vi "APLUS.vi"(8 "error in (no error)":errorcluster) -> (0 "error out":errorcluster, 2 "Stopped":bool)   [LabVIEW 2019]
uses:
  TypeDef/MB Modbus Command.ctl
  TypeDef/MISURE WT.ctl
  TypeDef/DEVICE NAME.ctl
  <vilib>/Utility/file.llb/Read Delimited Spreadsheet (string).vi
  <vilib>/Modbus/master/Create Master Instance (Serial).vi
  <vilib>/Modbus/master/Modbus Master.lvclass
panel:
  out "# elements in queue":i32
  out "tempo ciclo":u32
  out "element":string
  out "Iteration":i32
  out "STATO":string
  out "MISURE WT":T1
  out "Cluster 2":T2 {"Deviation from average of currents [I1,I2,I3]" format="%.2f"; "Deviation from average of voltages [U1,U2,U3]" format="%.2f"; "Maximum deviation from average of currents" format="%.2f"; "Maximum deviation from average of voltages" format="%.2f"; "Phase angle voltage U3-U1" format="%.2f"; "Phase angle voltage U2-U3" format="%.2f"; "Phase angle voltage U1-U2" format="%.2f"; "Average value of currents (I1+I2+I3)/3" format="%.2f"; "Average value of voltages (U1x+U2x+U3x)/3" format="%.2f"; "Load factor phase 3 (L3 – N)" format="%.2f"; "Load factor phase 2 (L2 – N)" format="%.2f"; "Load factor phase 1 (L1 – N)" format="%.2f"; "sign(Q)·(1 – abs(PF)), Load factor system" format="%.2f"; "Reactive power factor phase 1 (L3 – N)" format="%.2f"; "Reactive power factor phase 1 (L2 – N)" format="%.2f"; "Reactive power factor phase 1 (L1 – N)" format="%.2f"; "QF = Q / S, Reactive power factor system" format="%.2f"; "Power factor phase 3 (L3 – N)" format="%.2f"; "Power factor phase 2 (L2 – N)" format="%.2f"; "Power factor phase 1 (L1 – N)" format="%.2f"; "PF = P / S, Power factor system PF" format="%.2f"; "System frequency" format="%.2f"; "Apparent power phase 3 (L3 – N)" format="%.2f"; "Apparent power phase 2 (L2 – N)" format="%.2f"; "Apparent power phase 1 (L1 – N)" format="%.2f"; "Apparent power system S" format="%.2f"; "Reactive power phase 3 (L3 – N)" format="%.2f"; "Reactive power phase 2 (L2 – N)" format="%.2f"; "Reactive power phase 1 (L1 – N)" format="%.2f"; "Reactive power system (Q = Q1 + Q2 + Q3)" format="%.2f"; "Active power phase 3 (L3 – N)" format="%.2f"; "Active power phase 2 (L2 – N)" format="%.2f"; "Active power phase 1 (L1 – N)" format="%.2f"; "Active power system (P = P1 + P2 + P3)" format="%.2f"; "Bimetal current in phase L3" format="%.2f"; "Bimetal current in phase L2" format="%.2f"; "Bimetal current in phase L 1" format="%.2f"; "Bimet curr in balan load sys" format="%.2f"; "Neutral current" format="%.2f"; "Current in phase L3" format="%.2f"; "Current in phase L2" format="%.2f"; "Current in phase L1" format="%.2f"; "System current" format="%.2f"; "Zero displac volt 4w sys" format="%.2f"; "Voltage phase L3 to L1" format="%.2f"; "Voltage phase L2 to L3" format="%.2f"; "Voltage phase L1 to L2" format="%.2f"; "Voltage phase L3 to N" format="%.2f"; "Voltage phase L2 to N" format="%.2f"; "Voltage phase L1 to N" format="%.2f"; "System voltage" format="%.2f"}
  in  "milliseconds to wait":u32=20
  in  "Tab Control":T3(tab)
  in  "SETUP PORTA SERIALE":T4={"Porta COM"="COM2", "Baud Rate"=19200, "Parity"=0, "Flow Control"=0, "Timeout"=10000, "Mode"=enum."RTU", "Slave Address"=1} {"Flow Control" items=["None", "XON/XOFF", "RTS/CTS", "XON/XOFF & RTS/CTS", "DTR/DSR", "XON/XOFF & DTR/DSR"]; "Parity" items=["None", "Odd", "Even", "Mark", "Space"]}
  out "A primario":dbl format="%.20g"
  out "A secondario":dbl format="%.20g"
  out "Modalità misura":u16
  out "V primario":dbl format="%.20g"
  out "V secondario":dbl format="%.20g"
  out "freq":dbl format="%.20g"
  in  "READ REGISTER":bool
  in  "Modbus Command 2":T5={"Function Code"=3, "Starting Address"=2199, "Quantity"=12, "Data"=[], "Discrete"=[]} {"Function Code" items=["Read Coils"=1, "Read Discrete Inputs"=2, "Read Holding Registers"=3, "Read Input Registers"=4, "Write Single Coil"=5, "Write Single Register"=6, "Read Exception Status"=7, "Write Multiple Coils"=15, "Write Multiple Registers"=16]}
  in  "WRITE MODO MISURA":bool
  in  "Enum":T6(ring)
  in  "PRIM":sgl=20.0 format="%.12f"
  in  "WRITE A PRIM":bool
  in  "SEC":sgl=5.0 format="%.12f"
  in  "WRITE A SEC":bool
  out "Cluster":T7 {"Sys current" format="%.1p"; "Sys voltage" format="%.1p"; "Cosphi" format="%.1p"; "Frequenza" format="%.1p"; "Energia attiva -" format="%.2f"; "Energia attiva +" format="%.2f"; "Tensione FN3" format="%.1p"; "Tensione FN2" format="%.1p"; "Tensione FN1" format="%.1p"; "Papparente" format="%.2f"; "Preattiva" format="%.2f"; "Corrente 3" format="%.3f"; "Corrente 2" format="%.3f"; "TensioneL31" format="%.1p"; "TensioneL23" format="%.1p"; "TensioneL12" format="%.1p"; "Corrente" format="%.3f"; "Pattiva" format="%.2f"}
  out "error in (no error) 2":errorcluster
  # "2199"
  # "12"
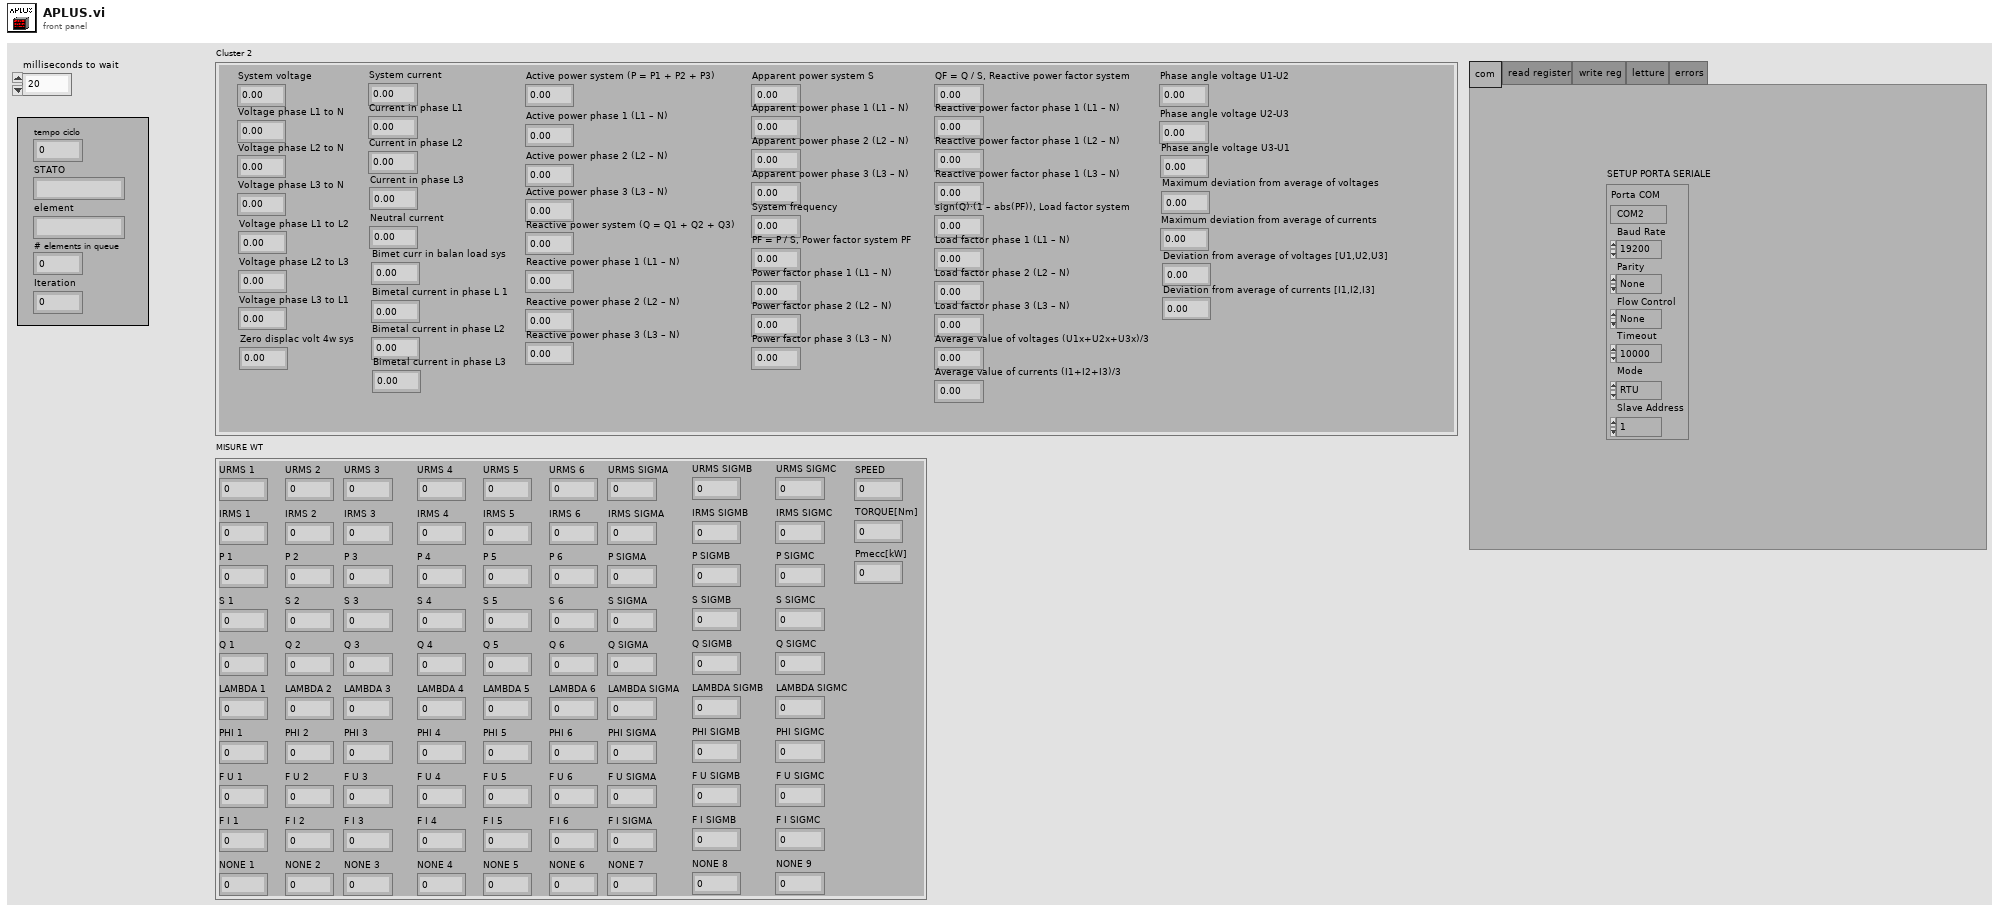
[diagram p1: front panel]
types:
  T1 = typedef "MISURE WT.ctl" = cluster{"URMS 1":dbl, "IRMS 1":dbl, "P 1":dbl, "S 1":dbl, "Q 1":dbl, "LAMBDA 1":dbl, "PHI 1":dbl, "F U 1":dbl, "F I 1":dbl, "NONE 1":dbl, "URMS 2":dbl, "IRMS 2":dbl, "P 2":dbl, "S 2":dbl, "Q 2":dbl, "LAMBDA 2":dbl, "PHI 2":dbl, "F U 2":dbl, "F I 2":dbl, "NONE 2":dbl, "URMS 3":dbl, "IRMS 3":dbl, "P 3":dbl, "S 3":dbl, "Q 3":dbl, "LAMBDA 3":dbl, "PHI 3":dbl, "F U 3":dbl, "F I 3":dbl, "NONE 3":dbl, "URMS 4":dbl, "IRMS 4":dbl, "P 4":dbl, "S 4":dbl, "Q 4":dbl, "LAMBDA 4":dbl, "PHI 4":dbl, "F U 4":dbl, "F I 4":dbl, "NONE 4":dbl, "URMS 5":dbl, "IRMS 5":dbl, "P 5":dbl, "S 5":dbl, "Q 5":dbl, "LAMBDA 5":dbl, "PHI 5":dbl, "F U 5":dbl, "F I 5":dbl, "NONE 5":dbl, "URMS 6":dbl, "IRMS 6":dbl, "P 6":dbl, "S 6":dbl, "Q 6":dbl, "LAMBDA 6":dbl, "PHI 6":dbl, "F U 6":dbl, "F I 6":dbl, "NONE 6":dbl, "URMS SIGMA":dbl, "IRMS SIGMA":dbl, "P SIGMA":dbl, "S SIGMA":dbl, "Q SIGMA":dbl, "LAMBDA SIGMA":dbl, "PHI SIGMA":dbl, "F U SIGMA":dbl, "F I SIGMA":dbl, "NONE 7":dbl, "URMS SIGMB":dbl, "IRMS SIGMB":dbl, "P SIGMB":dbl, "S SIGMB":dbl, "Q SIGMB":dbl, "LAMBDA SIGMB":dbl, "PHI SIGMB":dbl, "F U SIGMB":dbl, "F I SIGMB":dbl, "NONE 8":dbl, "URMS SIGMC":dbl, "IRMS SIGMC":dbl, "P SIGMC":dbl, "S SIGMC":dbl, "Q SIGMC":dbl, "LAMBDA SIGMC":dbl, "PHI SIGMC":dbl, "F U SIGMC":dbl, "F I SIGMC":dbl, "NONE 9":dbl, "SPEED":dbl, "TORQUE[Nm]":dbl, "Pmecc[kW]":dbl}
  T2 = cluster{"System voltage":dbl, "Voltage phase L1 to N":dbl, "Voltage phase L2 to N":dbl, "Voltage phase L3 to N":dbl, "Voltage phase L1 to L2":dbl, "Voltage phase L2 to L3":dbl, "Voltage phase L3 to L1":dbl, "Zero displac volt 4w sys":dbl, "System current":dbl, "Current in phase L1":dbl, "Current in phase L2":dbl, "Current in phase L3":dbl, "Neutral current":dbl, "Bimet curr in balan load sys":dbl, "Bimetal current in phase L 1":dbl, "Bimetal current in phase L2":dbl, "Bimetal current in phase L3":dbl, "Active power system (P = P1 + P2 + P3)":dbl, "Active power phase 1 (L1 – N)":dbl, "Active power phase 2 (L2 – N)":dbl, "Active power phase 3 (L3 – N)":dbl, "Reactive power system (Q = Q1 + Q2 + Q3)":dbl, "Reactive power phase 1 (L1 – N)":dbl, "Reactive power phase 2 (L2 – N)":dbl, "Reactive power phase 3 (L3 – N)":dbl, "Apparent power system S":dbl, "Apparent power phase 1 (L1 – N)":dbl, "Apparent power phase 2 (L2 – N)":dbl, "Apparent power phase 3 (L3 – N)":dbl, "System frequency":dbl, "PF = P / S, Power factor system PF":dbl, "Power factor phase 1 (L1 – N)":dbl, "Power factor phase 2 (L2 – N)":dbl, "Power factor phase 3 (L3 – N)":dbl, "QF = Q / S, Reactive power factor system":dbl, "Reactive power factor phase 1 (L1 – N)":dbl, "Reactive power factor phase 1 (L2 – N)":dbl, "Reactive power factor phase 1 (L3 – N)":dbl, "sign(Q)·(1 – abs(PF)), Load factor system":dbl, "Load factor phase 1 (L1 – N)":dbl, "Load factor phase 2 (L2 – N)":dbl, "Load factor phase 3 (L3 – N)":dbl, "Average value of voltages (U1x+U2x+U3x)/3":dbl, "Average value of currents (I1+I2+I3)/3":dbl, "Phase angle voltage U1-U2":dbl, "Phase angle voltage U2-U3":dbl, "Phase angle voltage U3-U1":dbl, "Maximum deviation from average of voltages":dbl, "Maximum deviation from average of currents":dbl, "Deviation from average of voltages [U1,U2,U3]":dbl, "Deviation from average of currents [I1,I2,I3]":dbl}
  T3 = enum32{"com", "read register", "write reg", "letture", "errors"}
  T4 = cluster{"Porta COM":string, "Baud Rate":u32, "Parity":u16, "Flow Control":u16, "Timeout":u32, "Mode":enum16{"RTU", "ASCII"}, "Slave Address":u8}
  T5 = typedef "MB Modbus Command.ctl" = cluster{"Function Code":u8, "Starting Address":u16, "Quantity":u16, "Data":u16[], "Discrete":bool[]}
  T6 = enum16{"SINGLE PH", "SPLIT PHASE", "3W,B", "3W,B,U12", "3W,B,U23", "3W,B,U31", "3W,U", "3W,U,ARON", "4W,B", "4W,U", "4W,U,OPEN_Y"}
  T7 = cluster{"Pattiva":dbl, "Corrente":dbl, "TensioneL12":dbl, "TensioneL23":dbl, "TensioneL31":dbl, "Corrente 2":dbl, "Corrente 3":dbl, "Preattiva":dbl, "Papparente":dbl, "Tensione FN1":dbl, "Tensione FN2":dbl, "Tensione FN3":dbl, "Energia attiva +":dbl, "Energia attiva -":dbl, "Frequenza":dbl, "Cosphi":dbl, "Sys voltage":dbl, "Sys current":dbl}
  T8 = typedef "DEVICE NAME.ctl" = enum16{"WATTMETRO", "APLUS", "PLC BANCO 1", "PLC RACK", "PLC BANCO 2", "PS", "NI cDAQ", "RESISTOMAT"}
  T9 = cluster{"Array of elements":cluster{"String":string, "variant":variant}[], "Single element":cluster{"String":string, "variant":variant}, "enque at\nopposite end (F)":bool, "no replications (F)":bool}
  T10 = enum16{"ALIGN -CENTER", "ALIGN -TOP LEFT", "ALIGN -AS IS", "ALIGN -CUSTOM"}
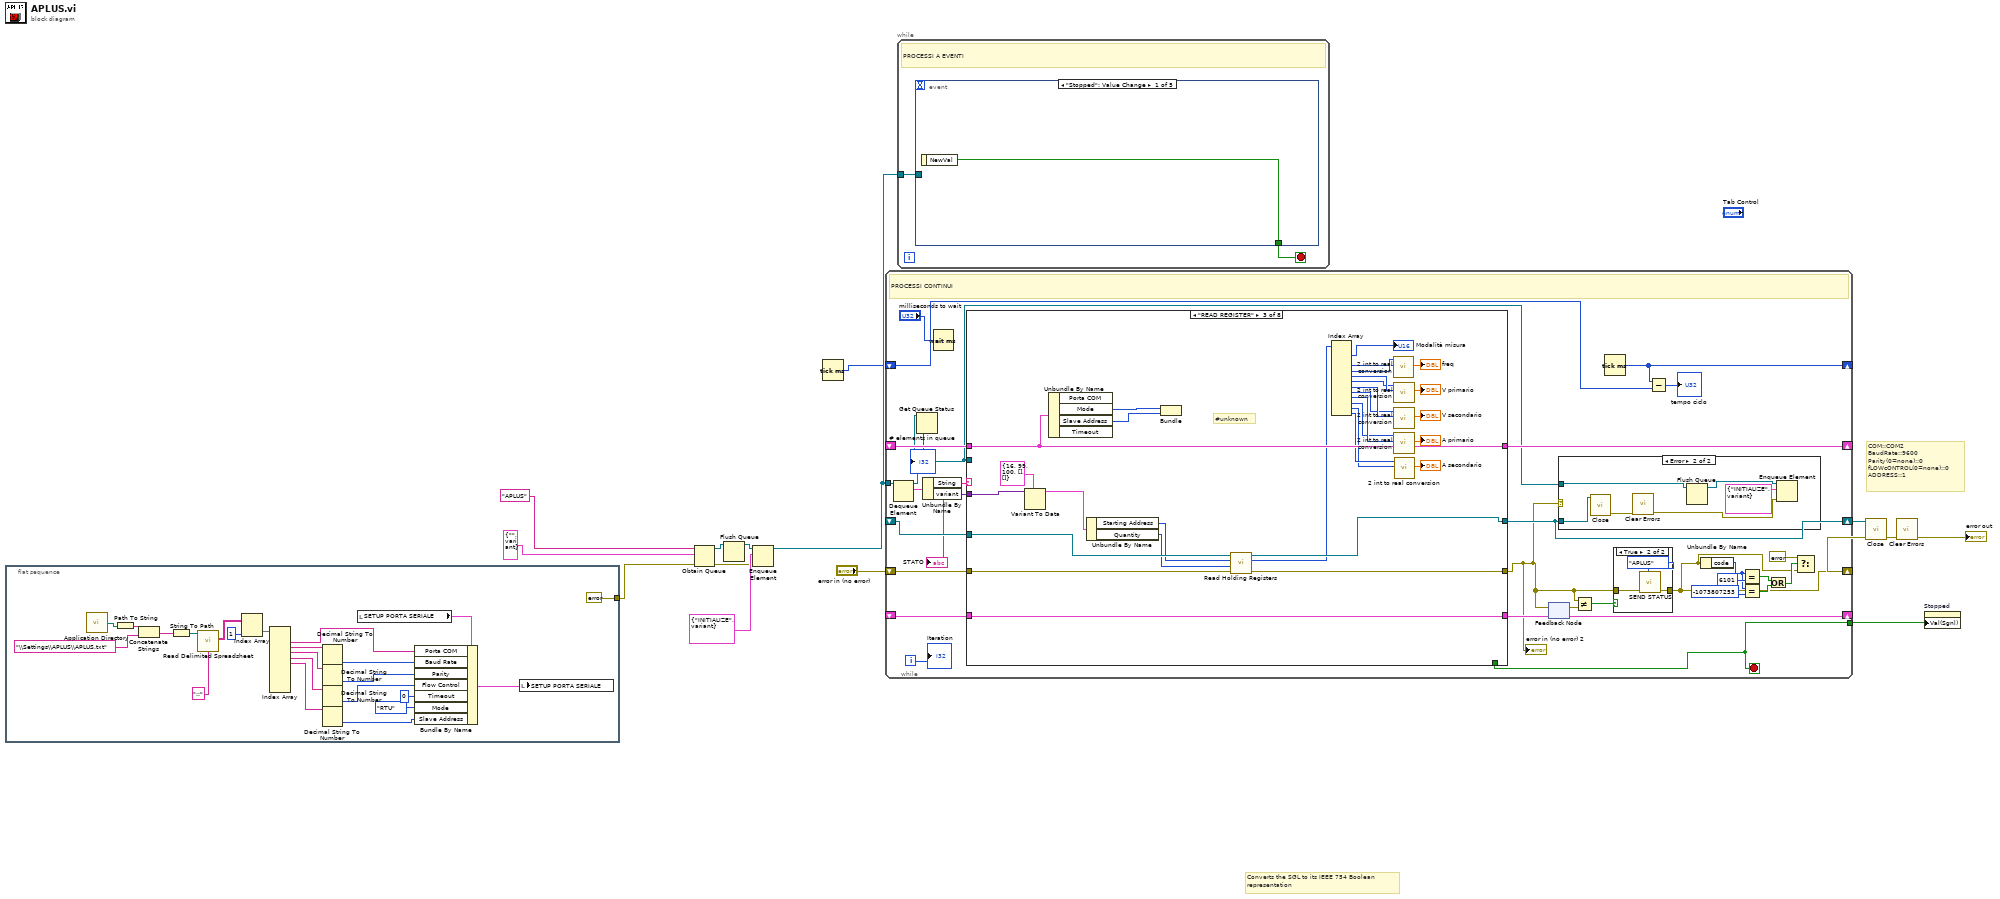
[diagram p0: block diagram]
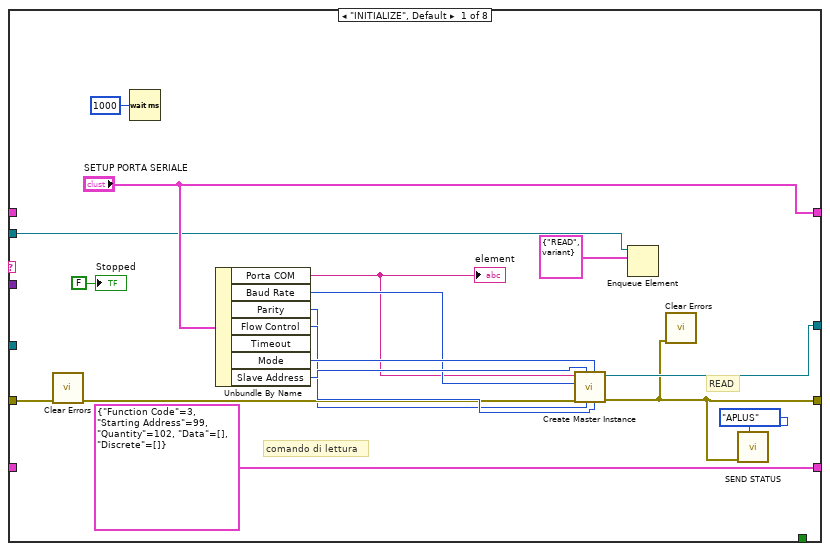
[diagram p4: hidden frame]
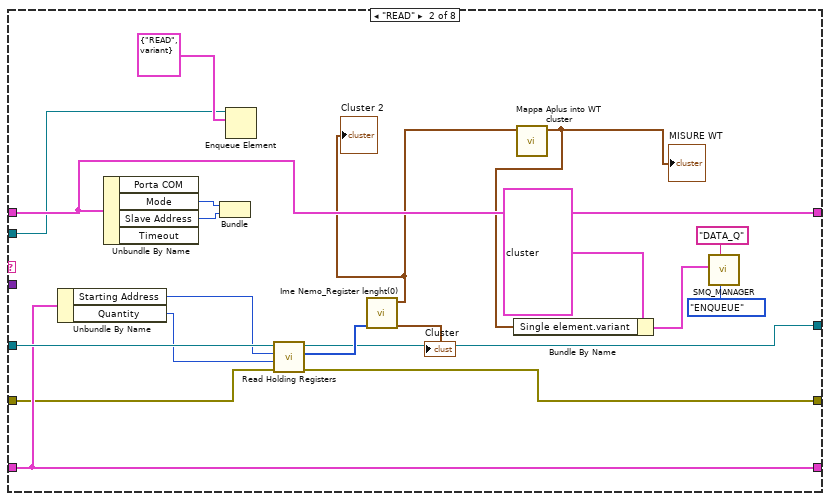
[diagram p5: hidden frame]
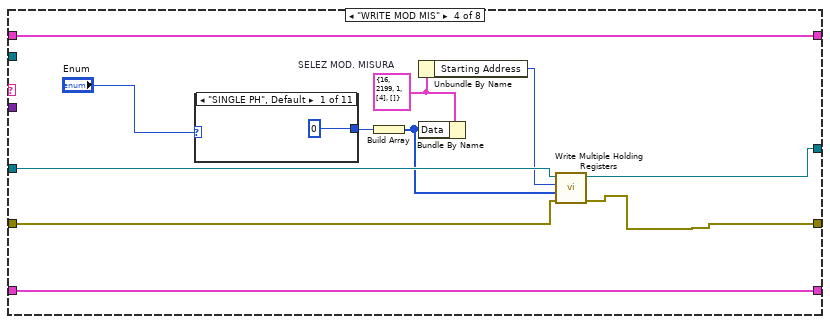
[diagram p6: hidden frame]
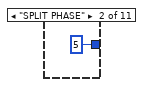
[diagram p7: hidden frame]
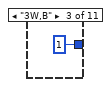
[diagram p8: hidden frame]
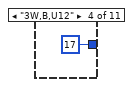
[diagram p9: hidden frame]
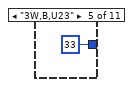
[diagram p10: hidden frame]
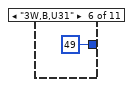
[diagram p11: hidden frame]
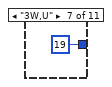
[diagram p12: hidden frame]
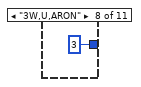
[diagram p13: hidden frame]
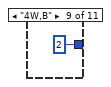
[diagram p14: hidden frame]
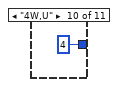
[diagram p15: hidden frame]
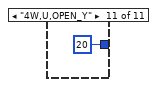
[diagram p16: hidden frame]
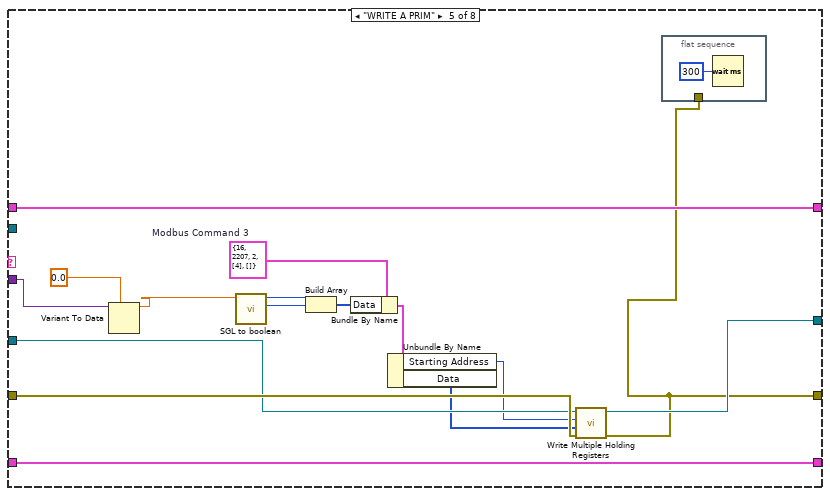
[diagram p17: hidden frame]
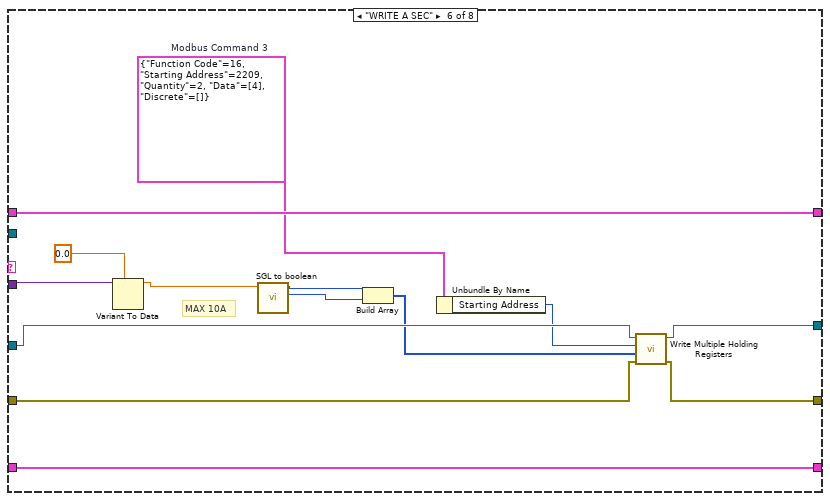
[diagram p18: hidden frame]
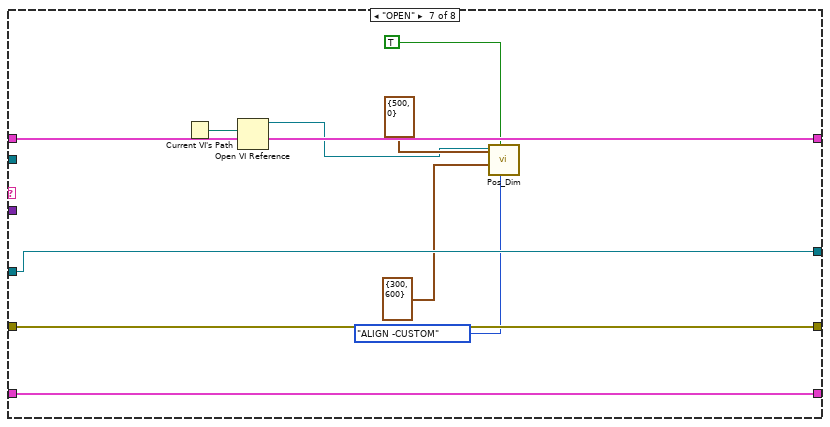
[diagram p19: hidden frame]
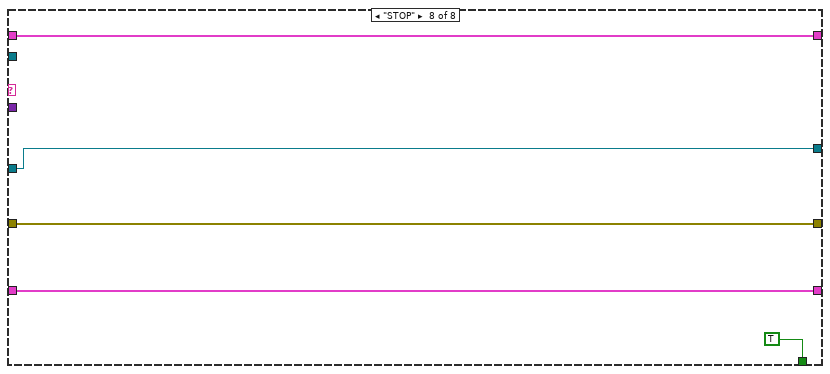
[diagram p20: hidden frame]
diagram:
  # "COM::COM2\nBaudRate::9600\nParity(0=none)::0\nfLOWcONTROL(0=none)::0\nADDRESS::1"
  # "Converts the SGL to its IEEE 754 Boolean \nrepresentation"
  n1 = flat-sequence {
    tunnel: [errorcluster {"status"=FALSE, "code"=0, "source"=""} ("error out")] -> w2
    frame #0 {
      n2 = call <vilib>:"Application Directory.vi"() -> ("Application Directory"=w26:path)
      n3 = Path To String(path=w26) -> (string=w27:string)
      n4 = Concatenate Strings(w27, "\\Settings\\APLUS\\APLUS.txt" ("string")) -> (w29:string)
      n5 = String To Path(string=w29) -> (path=w30:path)
      n6 = call-poly <vilib>:"Read Delimited Spreadsheet.vi"("file path (dialog if empty)"=w30, "delimiter (\\t)"="::" ("delimiter (\\t)")) -> ("all rows"=w31:string[][])  [unwired: 8 in, 5 out]
      n7 = Index Array(array=w31, index (col)=1 ("disabled index (col)")) -> (element=w33:string[])  [unwired: 1 in]
      n8 = Index Array(array=w33) -> (element #1=w22:string, element #2=w34:string, element #3=w35:string, element #4=w36:string, element #5=w37:string)  [unwired: 10 in, 5 out]
      n9 = Decimal String To Number(string=w34) -> (number=w21:i32)  [unwired: 2 in, 1 out]
      n10 = Decimal String To Number(string=w35) -> (number=w20:i32)  [unwired: 2 in, 1 out]
      n11 = Decimal String To Number(string=w36) -> (number=w19:i32)  [unwired: 2 in, 1 out]
      n12 = Decimal String To Number(string=w37) -> (number=w17:i32)  [unwired: 2 in, 1 out]
      n13 = local read "SETUP PORTA SERIALE"() -> (w24:T4)
      n14 = Bundle By Name(cluster=w24, "Porta COM"=w22, "Baud Rate"=w21, "Parity"=w20, "Flow Control"=w19, "Timeout"=u32 0, "Mode"=enum16{"RTU", "ASCII"}."RTU", "Slave Address"=w17) -> (w23:T4)
      n15 = local write "SETUP PORTA SERIALE"(w23) -> ()
    }
  }
  n16 = Obtain Queue(name (unnamed)="APLUS", element data type=cluster{"String":string, "variant":variant} {"String"="", "variant"=variant} ("element"), error in (no error)=w2) -> (queue out=w4:refnum<queue>, error out=w6:errorcluster)  [unwired: 2 in, 1 out]
  n17 = Flush Queue(queue=w4) -> (queue out=w3:refnum<queue>)  [unwired: 1 in, 2 out]
  n18 = Enqueue Element(queue=w3, element=cluster{"String":string, "variant":variant} {"String"="INITIALIZE", "variant"=variant}, error in (no error)=w6) -> (queue out=w13:refnum<queue>)  [unwired: 1 in, 2 out]
  n19 = Tick Count (ms)() -> (millisecond timer value=w1:u32)
  n20 = while {
    shift-right: [w47] -> w11
    shift-left: "error in (no error)" -> [w68]
    tunnel: w13 -> [w52]
    tunnel: [w48] -> w14
    shift-right: [w54] -> _
    shift-left: _ -> [w66]
    shift-right: [w65] -> _
    shift-left: _ -> [w64]
    shift-right: [w53] -> w12
    shift-left: _ -> [w55]
    shift-right: [w46] -> _
    shift-left: w1 -> [w45]
    i -> [w63]
    stop <- w48 stop-if-true
    # "PROCESSI CONTINUI"
    n21 = Dequeue Element(queue=w52) -> (queue out=w43:refnum<queue>, element=w51:cluster{"String":string, "variant":variant})  [unwired: 2 in, 2 out]
    n22 = Get Queue Status(queue=w43) -> (# elements in queue=→"# elements in queue":i32)  [unwired: 2 in, 7 out]
    n23 = Unbundle By Name(w51) -> ("String"=w49:string, "variant"=w50:variant)
    "STATO" <- w49
    n24 = Wait (ms)(milliseconds to wait="milliseconds to wait") -> ()  [unwired: 1 out]
    n25 = case shown="\"READ REGISTER\"" w49 {
      tunnel: [_ _ _ _ _ _ _ TRUE] -> w48
      tunnel: w68 -> [w84 w105 w123 w153 w177 w194 w208 w212]
      tunnel: [w79 w104 w122 w147 w171 w193 w208 w212] -> w40
      tunnel: w50 -> [_ _ w144 _ w170 w186 _ _]
      tunnel: w64 -> [_ w108 w145 w156 w183 w198 w206 w210]
      tunnel: ["SETUP PORTA SERIALE" w115 w140 w155 w181 w197 w207 w211] -> w54
      tunnel: w66 -> [_ w115 w140 w155 w181 w197 w207 w211]
      tunnel: [T5 {"Function Code"=3, "Starting Address"=99, "Quantity"=102, "Data"=[], "Discrete"=[]} ("Modbus Command") w108 w145 w156 w183 w198 w206 w210] -> w65
      tunnel: w43 -> [w91 w111 _ _ _ _ _ _]
      tunnel: [w85 w106 w120 w151 w175 w191 w205 w209] -> w53
      tunnel: w55 -> [_ w109 w121 w152 w176 w192 w205 w209]
      frame "INITIALIZE", Default {
        # "comando di lettura"
        # "READ"
        n26 = call <vilib>:"Clear Errors.vi"("error in (no error)"=w84) -> ("error out"=w83:errorcluster)  [unwired: 5 in, 1 out]
        n27 = Wait (ms)(milliseconds to wait=u32 1000) -> ()  [unwired: 1 out]
        n28 = Unbundle By Name("SETUP PORTA SERIALE") -> ("Porta COM"=w82:string, "Baud Rate"=w87:u32, "Parity"=w81:u16, "Flow Control"=w86:u16, "Mode"=w88:enum16{"RTU", "ASCII"}, "Slave Address"=w89:u8)  [unwired: 1 out]
        "element" <- w82
        n29 = call-poly <vilib>:"Create Master Instance.vi"("flow control (None)"=w86, "serial type"=w88, "parity (Even)"=w81, "unit ID"=w89, "error in (no error)"=w83, "baud rate (9600)"=w87, "VISA resource name"=w82) -> ("error out"=w79:errorcluster, "serial master instance"=w85:refnum<class "Modbus Master.lvclass">)  [unwired: 3 in]
        n30 = Enqueue Element(queue=w91, element=cluster{"String":string, "variant":variant} {"String"="READ", "variant"=variant}) -> ()  [unwired: 2 in, 3 out]
        n31 = call <vilib>:"Clear Errors.vi"("error in (no error)"=w79) -> ()  [unwired: 5 in, 2 out]
        n32 = call "SEND STATUS.vi"("ELEMENT"=DEVICE_NAME."APLUS", "error in (no error)"=w79) -> ()  [unwired: 9 in, 1 out]
        "Stopped" <- FALSE ("Stop")
      }
      frame "READ" {
        n33 = Unbundle By Name(w108) -> ("Starting Address"=w103:u16, "Quantity"=w102:u16)
        n34 = Unbundle By Name(w115) -> ("Mode"=w114:enum16{"RTU", "ASCII"}, "Slave Address"=w113:u8)  [unwired: 2 out]
        n35 = Bundle("Mode"=w114, "Slave Address"=w113) -> ()  [unwired: 1 in, 1 out]
        n36 = Enqueue Element(queue=w111, element=cluster{"String":string, "variant":variant} {"String"="READ", "variant"=variant}) -> ()  [unwired: 2 in, 3 out]
        n37 = call-dynamic "Read Holding Registers.vi"("error in (no error)"=w105, "number of holding registers"=w102, "starting address"=w103, "Modbus master in"=w109) -> ("error out"=w104:errorcluster, "register values"=w107:u16[], "Modbus master out"=w106:refnum<class "Modbus Master.lvclass">)  [unwired: 5 in]
        n38 = call "Ime Nemo_Register lenght(0).vi"("Array U16"=w107) -> ("Cluster"=→"Cluster":T7, "Cluster 2"=w101:T2)  [unwired: 9 in]
        "Cluster 2" <- w101
        n39 = call "Mappa Aplus into WT cluster.vi"("Cluster in"=w101) -> ("MISURE WT"=w96:T1)  [unwired: 10 in]
        "MISURE WT" <- w96
        n40 = Bundle By Name(cluster=T9 {"Array of elements"=[], "Single element"={"String"="READ WT", "variant"=variant}, "enque at\nopposite end (F)"=FALSE, "no replications (F)"=FALSE} ("Enqueue cluster"), "Single element.variant"=w96) -> (w97:T9)
        n41 = call <userlib>:"SMQ_MANAGER.vi"("Function"=enum16{"INITIALIZE", "ENQUEUE", "STOP ALL"}."ENQUEUE", "Queue name"="DATA_Q", "Enqueue cluster"=w97) -> ()  [unwired: 8 in, 1 out]
      }
      frame "READ REGISTER" {
        # "#unknown"
        n42 = Variant To Data(type=T5 {"Function Code"=16, "Starting Address"=99, "Quantity"=100, "Data"=[], "Discrete"=[]} ("Modbus Command"), Variant=w144) -> (data=w119:T5)  [unwired: 1 in, 1 out]
        n43 = Unbundle By Name(w140) -> ("Mode"=w142:enum16{"RTU", "ASCII"}, "Slave Address"=w141:u8)  [unwired: 2 out]
        n44 = Unbundle By Name(w119) -> ("Starting Address"=w118:u16, "Quantity"=w117:u16)
        n45 = Bundle("Mode"=w142, "Slave Address"=w141) -> ()  [unwired: 1 in, 1 out]
        n46 = call-dynamic "Read Holding Registers.vi"("error in (no error)"=w123, "number of holding registers"=w117, "starting address"=w118, "Modbus master in"=w121) -> ("error out"=w122:errorcluster, "register values"=w116:u16[], "Modbus master out"=w120:refnum<class "Modbus Master.lvclass">)  [unwired: 5 in]
        n47 = Index Array(array=w116) -> (element #1=→"Modalità misura":u16, element #3=w124:u16, element #4=w125:u16, element #5=w129:u16, element #6=w128:u16, element #7=w136:u16, element #8=w135:u16, element #9=w133:u16, element #10=w132:u16, element #11=w130:u16, element #12=w131:u16)  [unwired: 12 in, 1 out]
        n48 = call "2 int to real conversion.vi"("MW 15 0 in"=w124, "MW 31 16 in"=w125) -> ("reale out"=→"freq":dbl)  [unwired: 7 in, 2 out]
        n49 = call "2 int to real conversion.vi"("MW 15 0 in"=w129, "MW 31 16 in"=w128) -> ("reale out"=→"V primario":dbl)  [unwired: 7 in, 2 out]
        n50 = call "2 int to real conversion.vi"("MW 15 0 in"=w136, "MW 31 16 in"=w135) -> ("reale out"=→"V secondario":dbl)  [unwired: 7 in, 2 out]
        n51 = call "2 int to real conversion.vi"("MW 15 0 in"=w133, "MW 31 16 in"=w132) -> ("reale out"=→"A primario":dbl)  [unwired: 7 in, 2 out]
        n52 = call "2 int to real conversion.vi"("MW 15 0 in"=w130, "MW 31 16 in"=w131) -> ("reale out"=→"A secondario":dbl)  [unwired: 7 in, 2 out]
      }
      frame "WRITE MOD MIS" {
        w149 = T5 {"Function Code"=16, "Starting Address"=2199, "Quantity"=1, "Data"=[4], "Discrete"=[]}  # SELEZ MOD. MISURA
        n53 = case shown="\"SINGLE PH\", Default" "Enum" {
          tunnel: [i8 0 ("Numeric 2") i8 5 ("Numeric 2") i8 1 ("Numeric 2") i8 17 ("Numeric 2") i8 33 ("Numeric 2") i8 49 ("Numeric 2") i8 19 ("Numeric 2") i8 3 ("Numeric 2") i8 2 ("Numeric 2") i8 4 ("Numeric 2") i8 20 ("Numeric 2")] -> w154
          frame "SINGLE PH", Default {
          }
          frame "SPLIT PHASE" {
          }
          frame "3W,B" {
          }
          frame "3W,B,U12" {
          }
          frame "3W,B,U23" {
          }
          frame "3W,B,U31" {
          }
          frame "3W,U" {
          }
          frame "3W,U,ARON" {
          }
          frame "4W,B" {
          }
          frame "4W,U" {
          }
          frame "4W,U,OPEN_Y" {
          }
        }
        n54 = Build Array(w154) -> (w150:i8[])
        n55 = Unbundle By Name(w149) -> ("Starting Address"=w148:u16)
        n56 = Bundle By Name(cluster=w149, "Data"=w150) -> ()  [unwired: 1 out]
        n57 = call-dynamic "Write Multiple Holding Registers.vi"("error in (no error)"=w153, "holding register values"=w150, "starting address"=w148, "Modbus master in"=w152) -> ("error out"=w147:errorcluster, "Modbus master out"=w151:refnum<class "Modbus Master.lvclass">)  [unwired: 6 in]
      }
      frame "WRITE A PRIM" {
        w178 = T5 {"Function Code"=16, "Starting Address"=2207, "Quantity"=2, "Data"=[4], "Discrete"=[]}  # Modbus Command 3
        n58 = Variant To Data(type=0.0, Variant=w170) -> (data=w169:dbl)  [unwired: 1 in, 1 out]
        n59 = call "SGL to boolean.vi"("Number"=w169) -> ("Numeric 2"=w179:u32, "Numeric"=w180:u32)  [unwired: 9 in]
        n60 = Build Array(w180, w179) -> (w182:u32[])
        n61 = Bundle By Name(cluster=w178, "Data"=w182) -> (w174:T5)
        n62 = Unbundle By Name(w174) -> ("Starting Address"=w173:u16, "Data"=w172:u16[])
        n63 = call-dynamic "Write Multiple Holding Registers.vi"("error in (no error)"=w177, "holding register values"=w172, "starting address"=w173, "Modbus master in"=w176) -> ("error out"=w171:errorcluster, "Modbus master out"=w175:refnum<class "Modbus Master.lvclass">)  [unwired: 6 in]
        n64 = flat-sequence {
          tunnel: w171 -> [_]
          frame #0 {
            n65 = Wait (ms)(milliseconds to wait=u32 300) -> ()  [unwired: 1 out]
          }
        }
      }
      frame "WRITE A SEC" {
        w189 = T5 {"Function Code"=16, "Starting Address"=2209, "Quantity"=2, "Data"=[4], "Discrete"=[]}  # Modbus Command 3
        # "MAX 10A"
        n66 = Variant To Data(type=0.0, Variant=w186) -> (data=w185:dbl)  [unwired: 1 in, 1 out]
        n67 = call "SGL to boolean.vi"("Number"=w185) -> ("Numeric 2"=w195:u32, "Numeric"=w196:u32)  [unwired: 9 in]
        n68 = Build Array(w196, w195) -> (w190:u32[])
        n69 = Unbundle By Name(w189) -> ("Starting Address"=w188:u16)
        n70 = call-dynamic "Write Multiple Holding Registers.vi"("error in (no error)"=w194, "holding register values"=w190, "starting address"=w188, "Modbus master in"=w192) -> ("error out"=w193:errorcluster, "Modbus master out"=w191:refnum<class "Modbus Master.lvclass">)  [unwired: 6 in]
      }
      frame "OPEN" {
        n71 = Current VI's Path() -> (path=w200:path)
        n72 = Open VI Reference(vi path=w200) -> (vi reference=w199:refnum<vi>)  [unwired: 1 in, 5 out]
        n73 = call "Pos_Dim.vi"("Mode"=T10."ALIGN -CUSTOM", "Open FP"=TRUE, "Size"=cluster{"right":i16, "bottom":i16} {"right"=300, "bottom"=600}, "Poistion"=cluster{"left":i16, "top":i16} {"left"=500, "top"=0}, "VIRefNum  IN"=w199) -> ()  [unwired: 2 in, 5 out]
      }
      frame "STOP" {
      }
    }
    "error in (no error) 2" <- w40
    n74 = feedback-in #1(w40) -> ()
    n75 = feedback #1() -> (w41:errorcluster)  [unwired: 1 in]
    n76 = case shown="Error" w40 {
      tunnel: w43 -> [_ w74]
      tunnel: w53 -> [_ w78]
      frame No Error {
      }
      frame Error {
        n77 = call-dynamic "Close.vi"("Modbus master in"=w78) -> ("error out"=w76:errorcluster)  [unwired: 10 in]
        n78 = call <vilib>:"Clear Errors.vi"("error in (no error)"=w76) -> ("error out"=w75:errorcluster)  [unwired: 5 in, 1 out]
        n79 = Flush Queue(queue=w74) -> (queue out=w73:refnum<queue>)  [unwired: 1 in, 2 out]
        n80 = Enqueue Element(queue=w73, element=cluster{"String":string, "variant":variant} {"String"="INITIALIZE", "variant"=variant}, error in (no error)=w75) -> ()  [unwired: 1 in, 3 out]
      }
    }
    n81 = Not Equal?(x=w40, y=w41) -> (x != y?=w39:bool)
    n82 = Tick Count (ms)() -> (millisecond timer value=w46:u32)
    n83 = case shown="True" w39 {
      tunnel: [w69 w71] -> w47
      tunnel: w40 -> [w69 w70]
      frame False {
      }
      frame True {
        n84 = call "SEND STATUS.vi"("ELEMENT"=DEVICE_NAME."APLUS", "error in (no error)"=w70) -> ("error out"=w71:errorcluster)  [unwired: 9 in]
      }
    }
    n85 = Subtract(x=w46, y=w45) -> (x-y=→"tempo ciclo":u32)
    n86 = Unbundle By Name(w47) -> ("code"=w59:i32)
    n87 = Equal?(x=w59, y=6101) -> (x = y?=w60:bool)
    n88 = Equal?(x=w59, y=-1073807253) -> (x = y?=w57:bool)
    n89 = Or(x=w60, y=w57) -> (x .or. y?=w56:bool)
    n90 = Select(t=errorcluster {"status"=FALSE, "code"=0, "source"=""}, s=w56, f=w47) -> ()  [unwired: 1 out]
    "Iteration" <- w63
  }
  n91 = while {
    tunnel: w13 -> [w214]
    stop <- w215 stop-if-true
    # "PROCESSI A EVENTI"
    n92 = event shown="[0] \"Stopped\": Value Change" {
      selector: _ -> [_ _ _ _ _]
      dyn-events: _ -> [_ _ _ _ _]
      timeout: _ -> [_ _ _ _ _]
      tunnel: [w216 _ _ _ _] -> w215
      tunnel: w214 -> [_ w217 w224 w228 w235]
      event "Stopped": Value Change {
        n93 = event-data() -> ("NewVal"=w216:bool)  [unwired: 1 in]
      }
      event "READ REGISTER": Value Change {
        n94 = event-data() -> ("NewVal"=w218:bool)  [unwired: 1 in]
        n95 = case shown="True" w218 {
          tunnel: w217 -> [_ w223]
          frame False {
          }
          frame True {
            n96 = To Variant(anything="Modbus Command 2") -> (Variant=w220:variant)
            n97 = Bundle By Name(cluster=cluster{"String":string, "variant":variant} {"String"="READ REGISTER", "variant"=variant} ("element"), "variant"=w220) -> (w219:cluster{"String":string, "variant":variant})
            n98 = Enqueue Element(queue=w223, element=w219) -> ()  [unwired: 2 in, 3 out]
          }
        }
      }
      event "WRITE MODO MISURA": Value Change {
        n99 = event-data() -> ("NewVal"=w225:bool)  [unwired: 1 in, 1 out]
        n100 = case shown="True" w225 {
          tunnel: w224 -> [_ w227]
          frame False {
          }
          frame True {
            n101 = Enqueue Element(queue=w227, element=cluster{"String":string, "variant":variant} {"String"="WRITE MOD MIS", "variant"=variant}) -> ()  [unwired: 2 in, 3 out]
          }
        }
      }
      event "WRITE A PRIM": Value Change {
        n102 = event-data() -> ("NewVal"=w229:bool)  [unwired: 1 in, 1 out]
        n103 = case shown="True" w229 {
          tunnel: w228 -> [_ w233]
          frame False {
          }
          frame True {
            n104 = Bundle By Name(cluster=cluster{"String":string, "variant":variant} {"String"="WRITE A PRIM", "variant"=variant} ("element"), "variant"="PRIM") -> (w231:cluster{"String":string, "variant":variant})
            n105 = Enqueue Element(queue=w233, element=w231) -> ()  [unwired: 2 in, 3 out]
          }
        }
      }
      event "WRITE A SEC": Value Change {
        n106 = event-data() -> ("NewVal"=w234:bool)  [unwired: 1 in, 1 out]
        n107 = case shown="True" w234 {
          tunnel: w235 -> [_ w239]
          frame False {
          }
          frame True {
            n108 = Bundle By Name(cluster=cluster{"String":string, "variant":variant} {"String"="WRITE A SEC", "variant"=variant} ("element"), "variant"="SEC") -> (w237:cluster{"String":string, "variant":variant})
            n109 = Enqueue Element(queue=w239, element=w237) -> ()  [unwired: 2 in, 3 out]
          }
        }
      }
    }
  }
  n110 = call-dynamic "Close.vi"("error in (no error)"=w11, "Modbus master in"=w12) -> ("error out"=w10:errorcluster)  [unwired: 9 in]
  n111 = call <vilib>:"Clear Errors.vi"("error in (no error)"=w10) -> ("error out"=→"error out":errorcluster)  [unwired: 5 in, 1 out]
  n112 = property on="Stopped" class="Bool (strict)"("Val(Sgnl)"=w14) -> ()  [unwired: 2 in, 2 out]
